vi "Trigger Comm Event for Listen.vi"(8 "error in (no error)":errorcluster, 11 "CIFCorePlugin in":refnum<class "CIFCorePlugin.lvclass">) -> (0 "error out":errorcluster)   [LabVIEW 2021, in "CIFCorePlugin.lvclass"]
doc: "Trigger the Listen event for new communications. If the plugin is in the listening mode this will cause it to trigger that a new communication has been passed via the OOB channels. The channel will be checked on a timeout, so this is not required but will cause faster response."
uses:
  CIFCorePlugin.lvclass
  CIFCorePlugin.lvclass/CIFCorePlugin.ctl
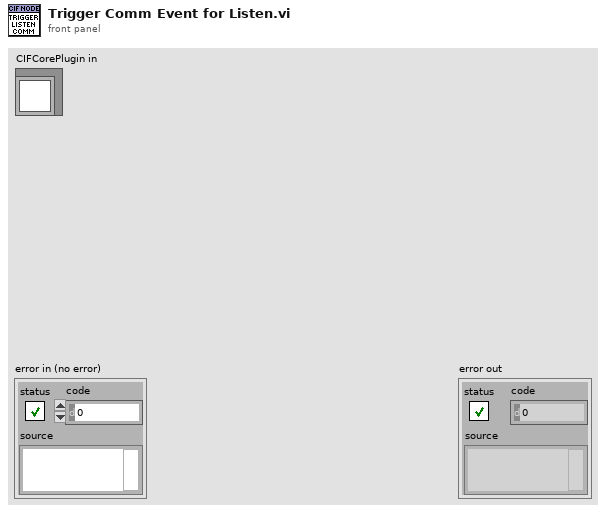
[diagram p1: front panel]
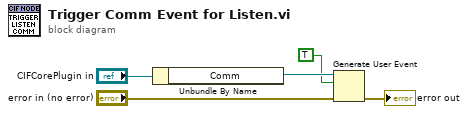
[diagram p0: block diagram]
diagram:
  n1 = Unbundle By Name("CIFCorePlugin in") -> ("Comm"=w2:refnum<user-event>)
  n2 = Generate User Event(user event=w2, event data cluster=TRUE ("event data"), error in="error in (no error)") -> (error out=→"error out":errorcluster)  [unwired: 1 in, 1 out]
